vi "FGV CalZustand.vi"(0 "CAL Zustand":u16, 5 "CG Eingang":u16, 9 "Aktion":T1) -> (14 "CAL Zustand FTIR":u16, 15 "CAL Zustand PMA":u16, 16 "CAL Zustand FID CH4":u16, 17 "CAL Zustand FID THC":u16, 19 "CG Eingang":u16)   [LabVIEW 2020, in "Auto Kalibrieren.lvlib"]
uses:
  Auto Kalibrieren.lvlib
  Aktion FGV CalZustand.ctl
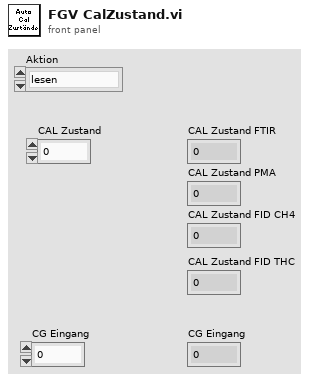
[diagram p1: front panel]
types:
  T1 = typedef "Auto Kalibrieren.lvlib/Aktion FGV CalZustand.ctl" = enum16{"lesen", "Cal FTIR", "Cal FID CH4", "Cal PMA", "init", "Cal FID THC", "THC CG Eingang"}
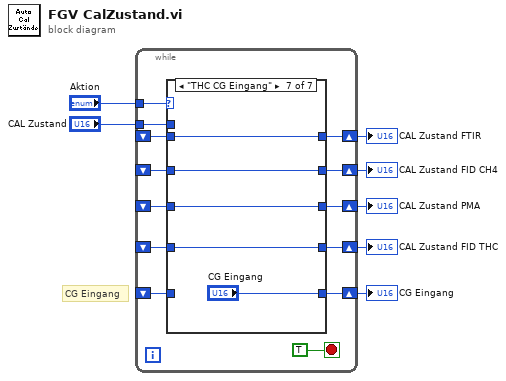
[diagram p0: block diagram]
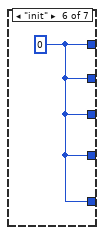
[diagram p7: hidden frame]
diagram:
  # "CG Eingang"
  n1 = while {
    tunnel: "Aktion" -> [w19]
    shift-right: [w18] -> w6
    shift-left: _ -> [w13]
    shift-right: [w17] -> w5
    shift-left: _ -> [w14]
    shift-right: [w16] -> w4
    shift-left: _ -> [w15]
    shift-right: [w12] -> w3
    shift-left: _ -> [w11]
    tunnel: "CAL Zustand" -> [w10]
    shift-right: [w8] -> w1
    shift-left: _ -> [w9]
    stop <- TRUE stop-if-true
    n2 = case shown="\"THC CG Eingang\"" w19 {
      tunnel: [w25 w30 w32 w40 w44 w46 w51] -> w18
      tunnel: [w24 w29 w35 w37 w45 w46 w50] -> w17
      tunnel: [w23 w28 w34 w39 w42 w46 w49] -> w16
      tunnel: w15 -> [w23 w28 w34 w39 _ _ w49]
      tunnel: w14 -> [w24 w29 w35 _ w45 _ w50]
      tunnel: w13 -> [w25 w30 _ w40 w44 _ w51]
      tunnel: [w22 w27 w33 w38 w43 w46 w48] -> w12
      tunnel: w11 -> [w22 _ w33 w38 w43 _ w48]
      tunnel: w10 -> [_ w27 w32 w37 w42 _ _]
      tunnel: w9 -> [w21 w26 w31 w36 w41 _ _]
      tunnel: [w21 w26 w31 w36 w41 w46 "CG Eingang"] -> w8
      frame "lesen", Default {
      }
      frame "Cal FID THC" {
      }
      frame "Cal FTIR" {
      }
      frame "Cal FID CH4" {
      }
      frame "Cal PMA" {
      }
      frame "init" {
        w46 = u16 0 ("CAL Zustand FTIR")
      }
      frame "THC CG Eingang" {
      }
    }
  }
  "CAL Zustand FTIR" <- w6
  "CAL Zustand FID CH4" <- w5
  "CAL Zustand PMA" <- w4
  "CAL Zustand FID THC" <- w3
  "CG Eingang" <- w1
